vi "Parallel Process Template (JKI-QSM).vi"() -> ()   [LabVIEW 2011, in "Messenging.lvlib" / "Parallel Process Template (JKI-QSM).lvclass"]
uses:
  Parallel Process Template (JKI-QSM).lvclass
  Interprocess Messenger/TextVarientMessage/Write VarMessage.vi
  Interprocess Messenger/VarMessage/VarMessage.lvclass
  Interprocess Messenger/TextVarientMessage/MSG.lvclass
  Parallel Process.lvclass
  Interprocess Messenger/TextVarientMessage/Write (no data).vi
  Interprocess Messenger/EventMessenger/EventMessenger.lvclass
  ObserverRegister/ObserverRegistry.lvclass
  Interprocess Messenger/ErrorMessage/Write ErrorMessage.vi
  Interprocess Messenger/ErrorMessage/ErrorMessage.lvclass
  Interprocess Messenger/TextVarientMessage/Reply (message).vi
panel:
  in  "Startup Message":refnum<class "MSG.lvclass">
  out "current time":timestamp
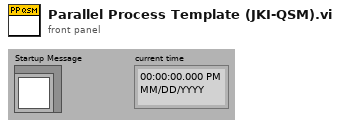
[diagram p1: front panel]
types:
  T1 = enum32{"invalid app kind", "Development System", "Run Time System", "Student Edition", "Embedded LabVIEW", "Evaluation", "Custom"}
  T2 = enum32{"Invalid", "Standard", "Closed", "Hidden", "Minimized", "Maximized"}
  T3 = cluster{"Core":cluster{"Current VI Reference":refnum<vi>, "Close Panel on Exit?":bool}, "Message":refnum<class "MSG.lvclass">, "事件注册引用句柄":refnum<event-registration>}
  T4 = cluster{"Current VI Reference":refnum<vi>, "Close Panel on Exit?":bool}
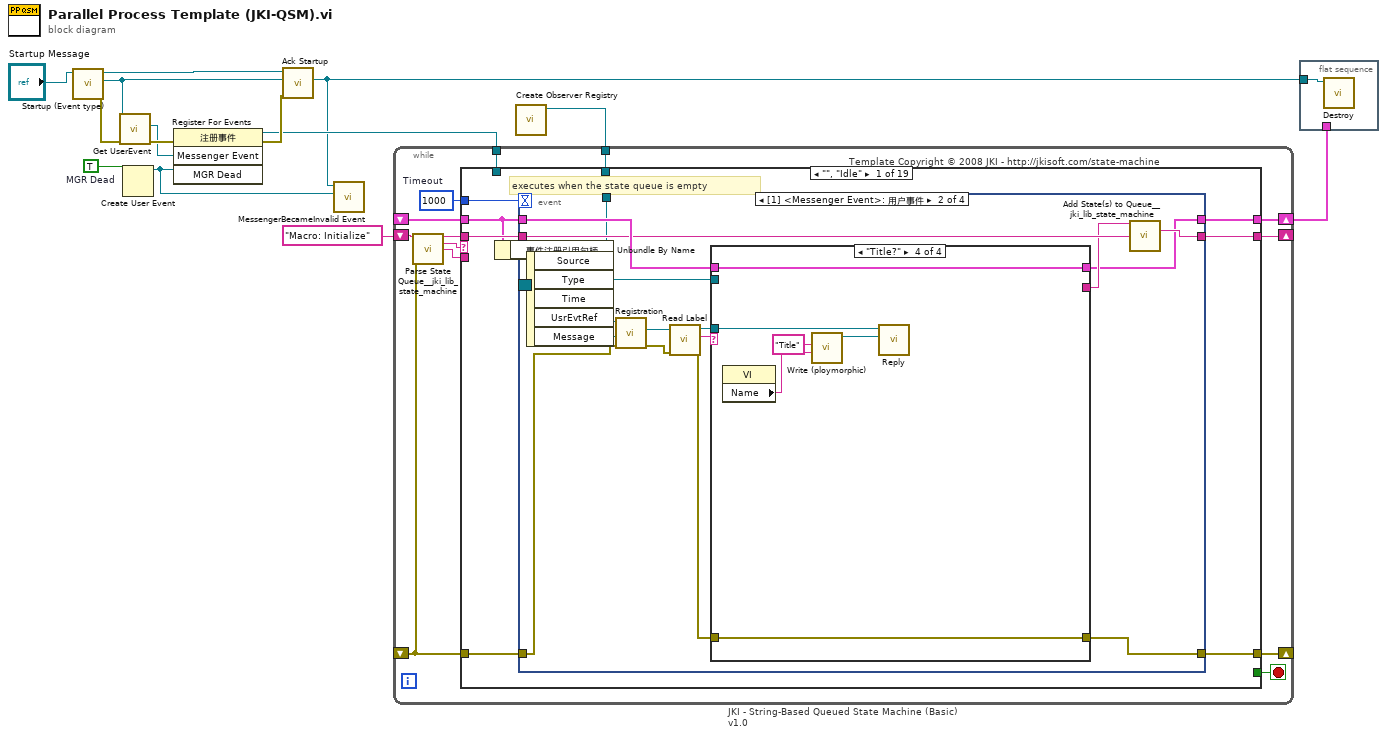
[diagram p0: block diagram]
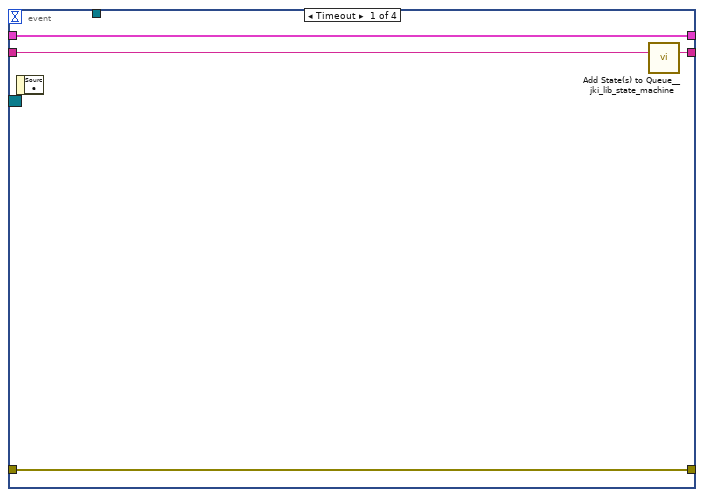
[diagram p2: hidden frame]
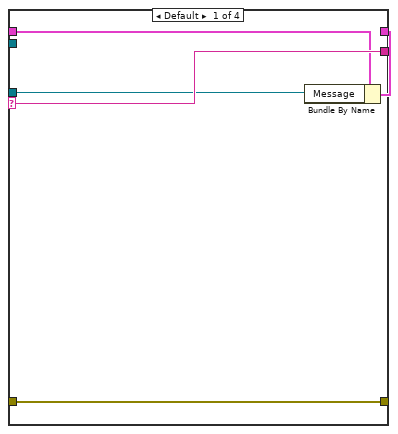
[diagram p3: hidden frame]
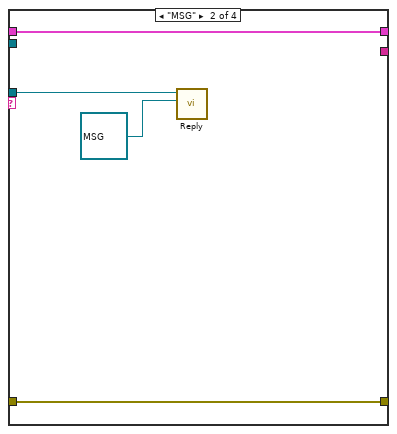
[diagram p4: hidden frame]
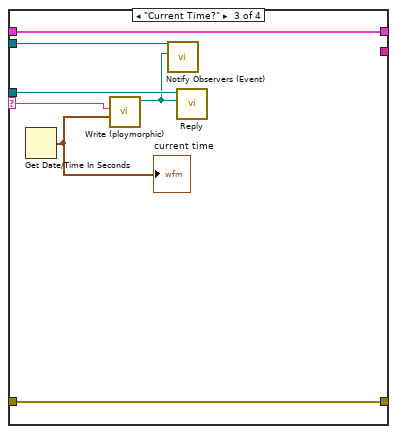
[diagram p5: hidden frame]
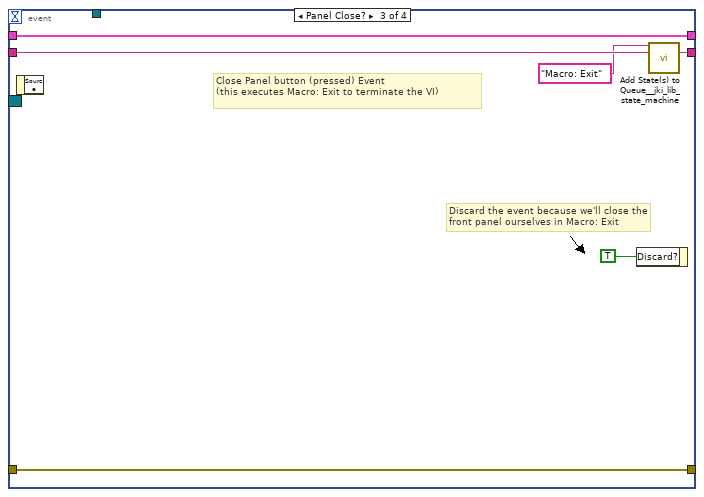
[diagram p6: hidden frame]
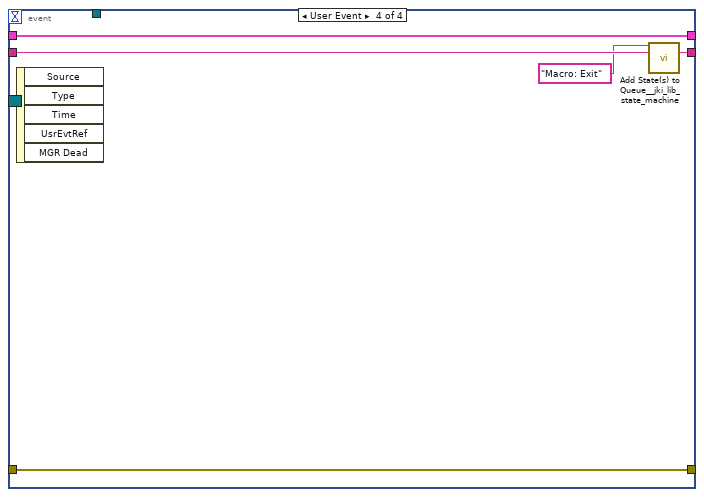
[diagram p7: hidden frame]
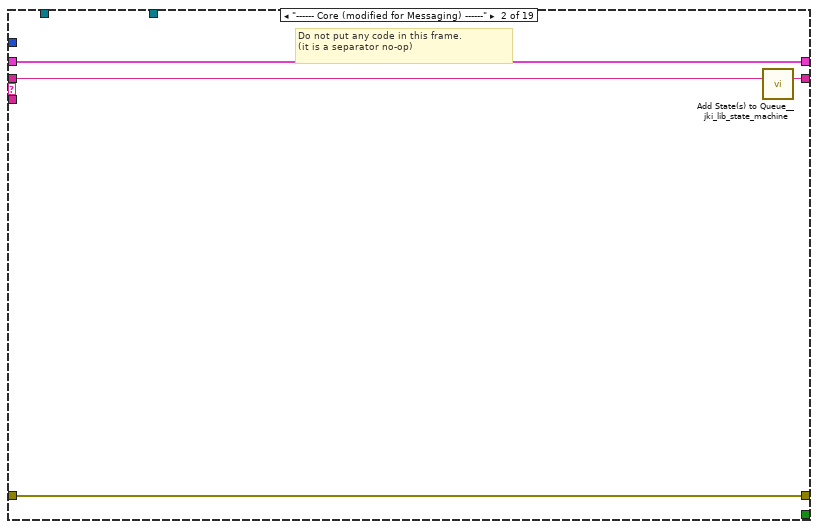
[diagram p8: hidden frame]
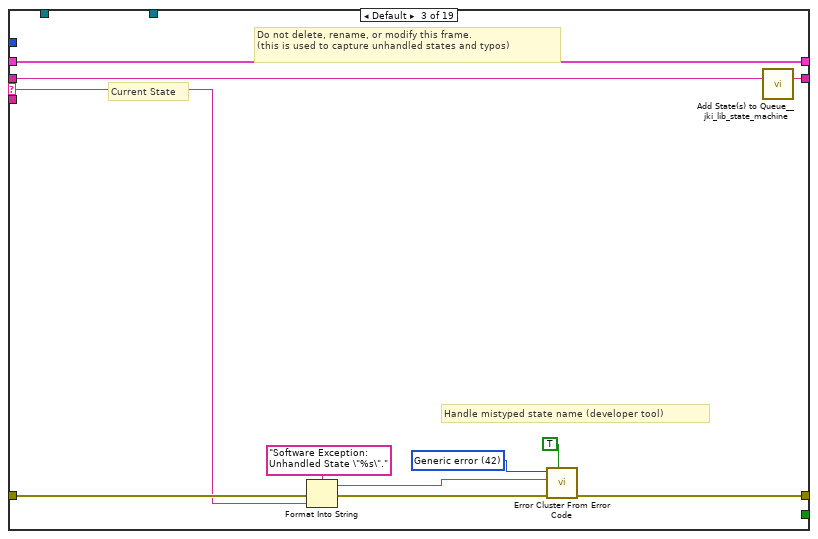
[diagram p9: hidden frame]
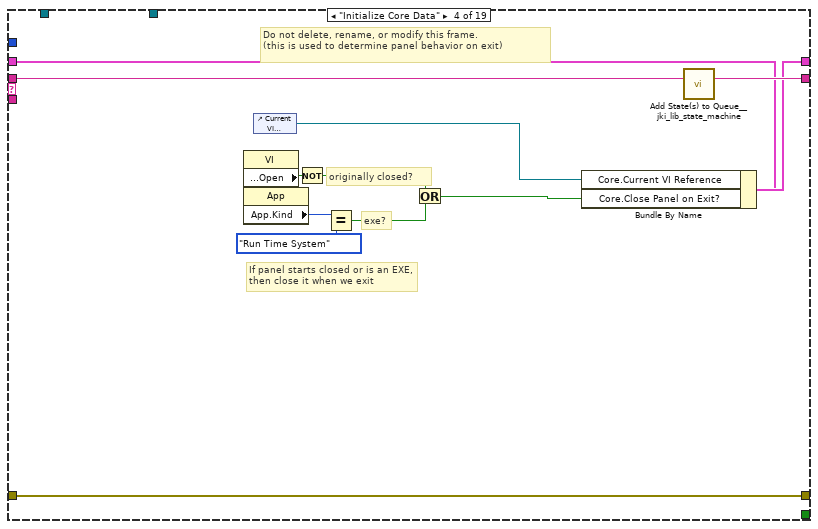
[diagram p10: hidden frame]
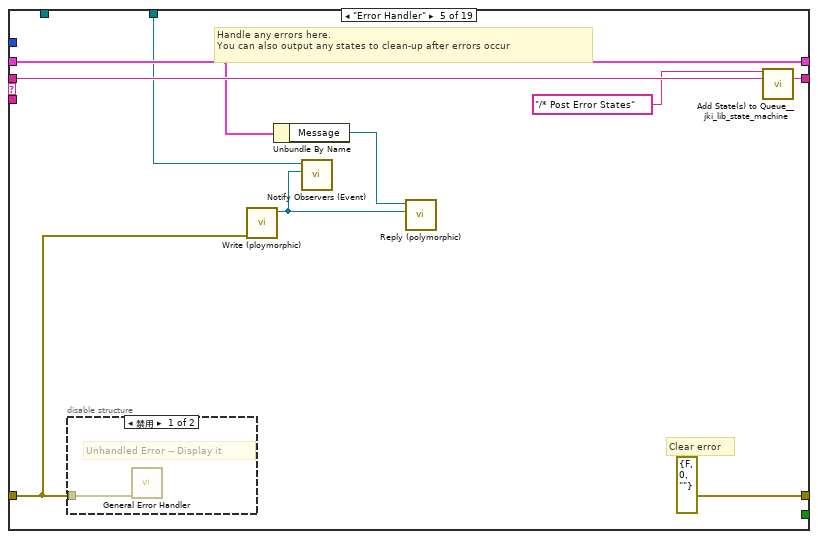
[diagram p11: hidden frame]
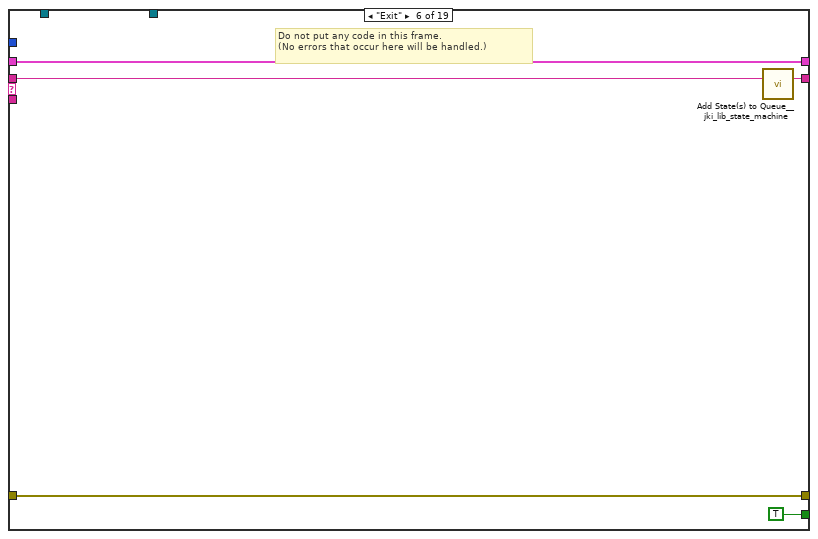
[diagram p13: hidden frame]
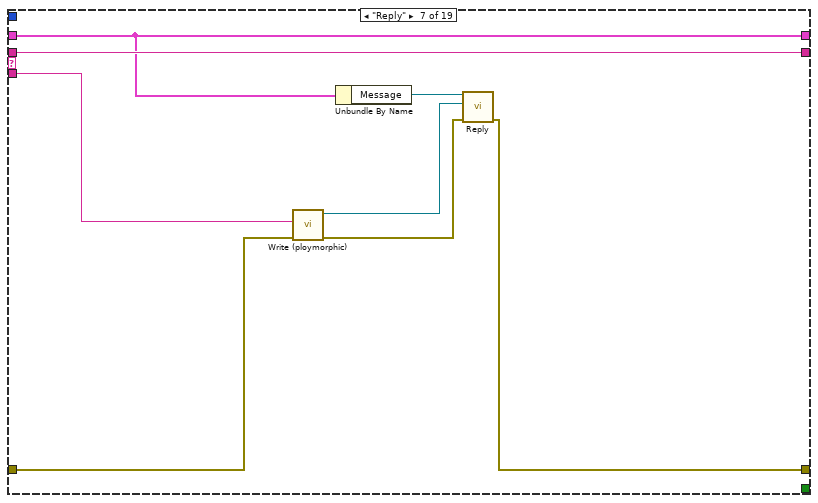
[diagram p14: hidden frame]
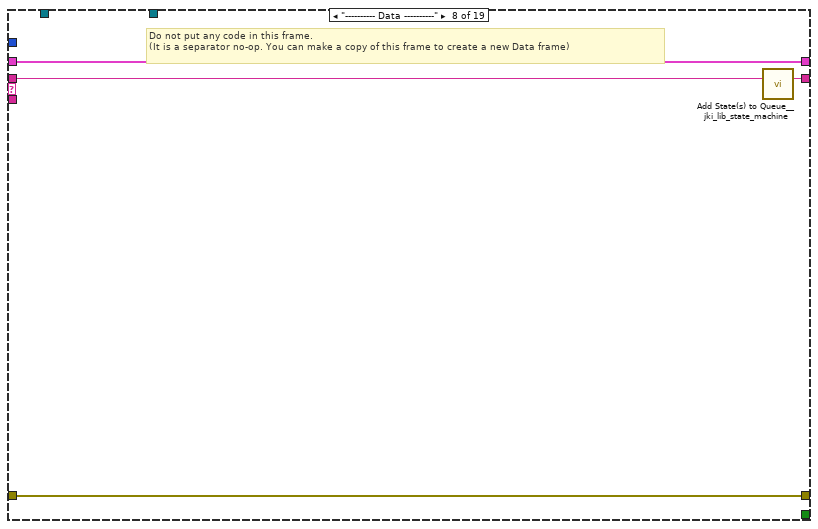
[diagram p15: hidden frame]
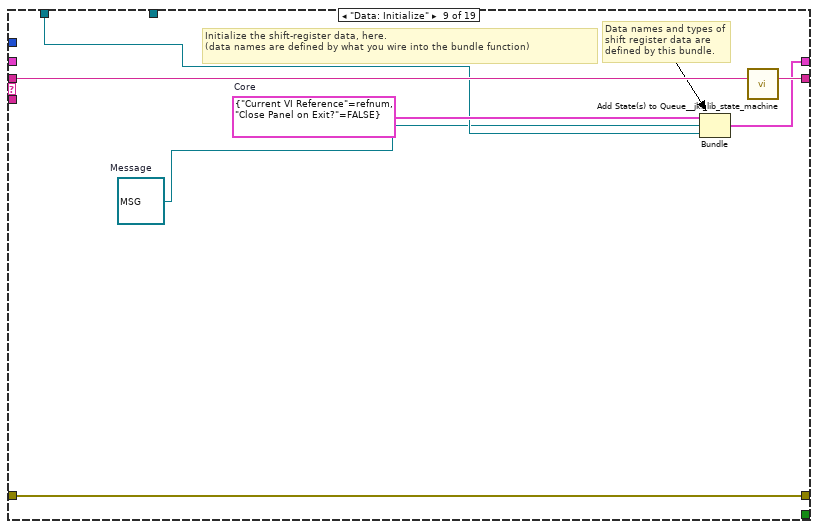
[diagram p16: hidden frame]
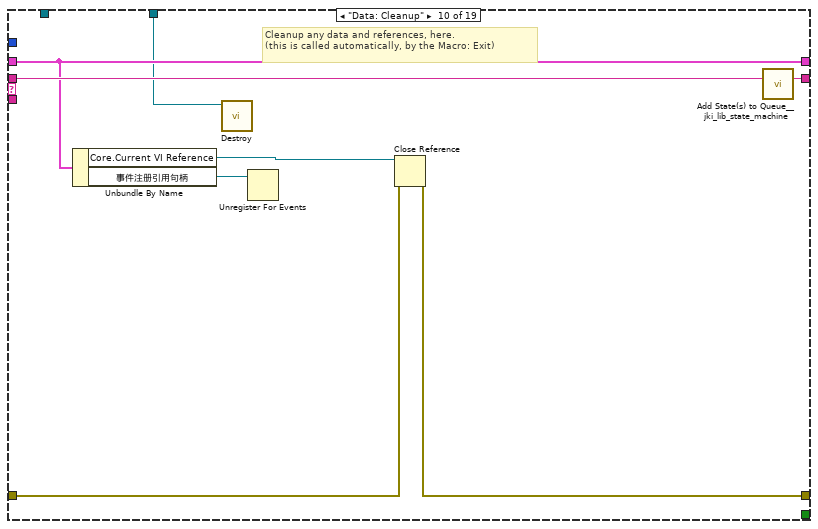
[diagram p17: hidden frame]
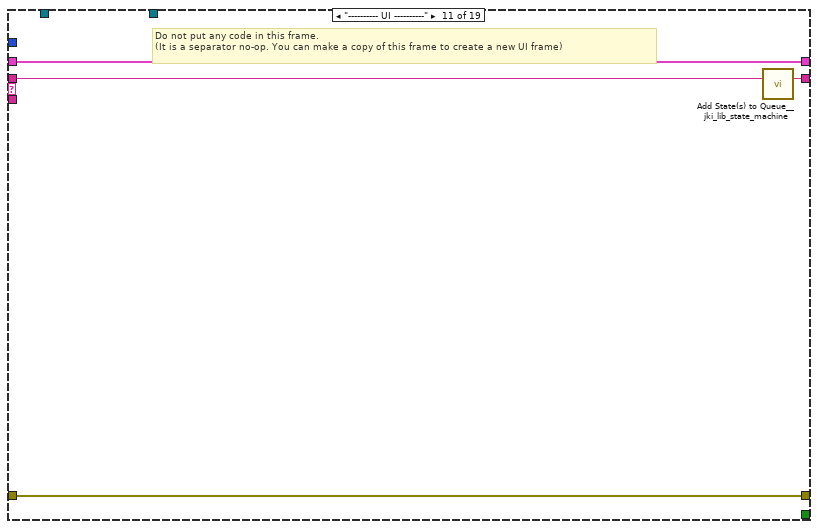
[diagram p18: hidden frame]
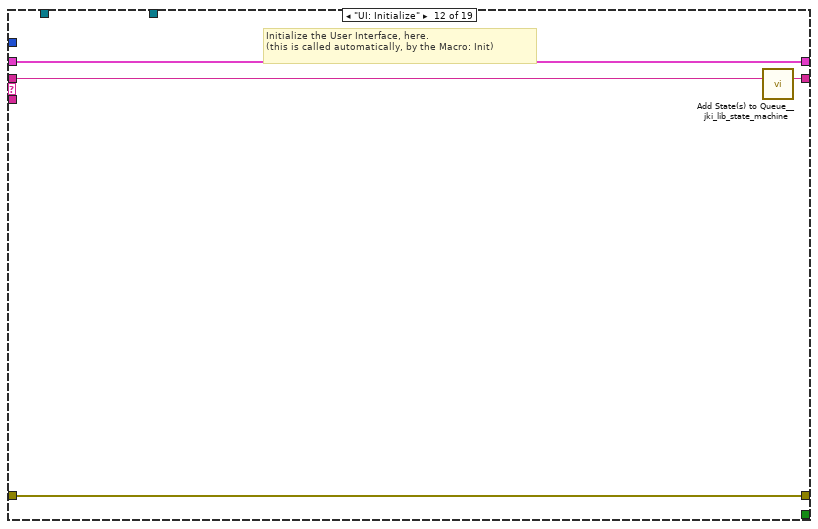
[diagram p19: hidden frame]
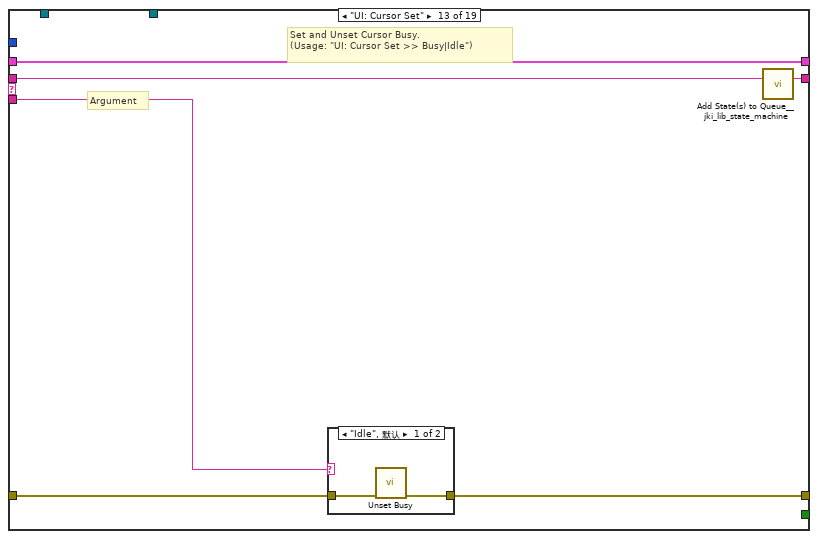
[diagram p20: hidden frame]
diagram:
  w8 = TRUE  # MGR Dead
  n1 = call "Startup (Event type).vi"("Startup Message"="Startup Message") -> ("error out"=w11:errorcluster, "Command Messenger out"=w13:refnum<class "EventMessenger.lvclass">, "Starup Message"=w12:refnum<class "MSG.lvclass">)  [unwired: 2 in, 6 out]
  n2 = call-dynamic "Get UserEvent.vi"("error in"=w11, "EventMessenger"=w13) -> ("error out"=w10:errorcluster, "Messenger Event"=w9:refnum<user-event>)  [unwired: 8 out]
  n3 = Create User Event(user event datatype=w8) -> (user event=w6:refnum<user-event>)  [unwired: 1 in, 1 out]
  n4 = register-events(error in=w10, w9, w6) -> (reference out=w5:refnum<event-registration>, error out=w7:errorcluster)  [unwired: 1 in]
  n5 = call "Ack Startup.vi"("error in"=w7, "Command Messenger"=w13, "Starup Message"=w12) -> ("Command Messenger"=w4:refnum<class "EventMessenger.lvclass">)  [unwired: 3 in, 5 out]
  n6 = call "MessengerBecameInvalid Event.vi"("MGR became Invalid"=w6, "Messenger"=w4) -> ()  [unwired: 1 in, 9 out]
  n7 = call "Create Observer Registry.vi"() -> ("ObsReg"=w1:refnum<class "ObserverRegistry.lvclass">)  [unwired: 1 in, 10 out]
  n8 = while "JKI - String-Based Queued State Machine (Basic) v1.0" {
    shift-right: [w20] -> w3
    shift-left: _ -> [w19]
    shift-right: [w23] -> _
    shift-left: _ -> [w17]
    shift-right: [w22] -> _
    shift-left: "Macro: Initialize" -> [w24]
    tunnel: w5 -> [w16]
    tunnel: w1 -> [w15]
    stop <- w21 stop-if-true
    w18 = 1000  # Timeout
    # "Template Copyright © 2008 JKI - http://jkisoft.com/state-machine"
    n9 = call <vilib>:"Parse State Queue__jki_lib_state_machine.vi"("State Queue"=w24, "Error In (no error)"=w17) -> ("Remaining States"=w26:string, "Current State"=w27:string, "Arguments"=w25:string)  [unwired: 1 in, 10 out]
    n10 = case shown="\"\", \"Idle\"" w27 {
      selector: w27 -> [_ _ w95 _ _ _ _ _ _ _ _ _ _ _ _ _ w215 _ _]
      tunnel: w26 -> [w36 w91 w98 w114 w123 w129 w137 w141 w148 w156 w160 w164 w170 w181 w207 w212 w225 w229 w233]
      tunnel: w25 -> [_ _ _ _ _ _ w130 _ _ _ _ _ w165 w175 _ _ _ _ _]
      tunnel: w19 -> [w30 w88 w94 w105 w119 w127 w133 w138 _ w151 w157 w162 w168 w177 w204 w209 w216 w226 w230]
      tunnel: [w34 w89 w92 w111 errorcluster {"status"=FALSE, "code"=0, "source"=""} ("error out") w126 w131 w139 w145 w152 w158 w161 w166 w178 w205 w210 w223 w227 w231] -> w23
      tunnel: w17 -> [w33 w89 w99 w111 w118 w126 w132 w139 w145 w153 w158 w161 w167 w179 w205 w210 w223 w227 w231]
      tunnel: [w35 w90 w97 w113 w122 w128 w137 w140 w147 w155 w159 w163 w169 w180 w206 w211 w224 w228 w232] -> w22
      tunnel: [_ _ _ _ _ TRUE _ _ _ _ _ _ _ _ _ _ _ _ _] -> w21
      tunnel: [w32 w88 w94 w112 w119 w127 w133 w138 w146 w151 w157 w162 w168 w177 w204 w209 w216 w226 w230] -> w20
      tunnel: w18 -> [w31 _ _ _ _ _ _ _ _ _ _ _ _ _ _ _ _ _ _]
      tunnel: w16 -> [_ _ _ _ _ _ _ _ w143 _ _ _ _ _ _ _ _ _ _]
      tunnel: w15 -> [w28 _ _ _ w116 _ _ _ _ w149 _ _ _ _ _ _ w213 _ _]
      frame "", "Idle" {
        # "executes when the state queue is empty"
        n11 = Unbundle By Name(w30) -> ("事件注册引用句柄"=w29:refnum<event-registration>)
        n12 = event shown="[1] <Messenger Event>: 用户事件" {
          selector: w29 -> [_ _ _ _]
          dyn-events: _ -> [_ _ _ _]
          timeout: w31 -> [_ _ _ _]
          tunnel: w36 -> [w40 w50 w82 w87]
          tunnel: [w39 w54 w81 w86] -> w35
          tunnel: w30 -> [w37 w53 w79 w84]
          tunnel: [w38 w47 w80 w85] -> w34
          tunnel: w33 -> [w38 w43 w80 w85]
          tunnel: [w37 w48 w79 w84] -> w32
          tunnel: w28 -> [_ w41 _ _]
          event Timeout {
            n13 = event-data() -> ()  [unwired: 2 out]
            n14 = call <vilib>:"Add State(s) to Queue__jki_lib_state_machine.vi"("State(s) in (\"\")"=w40) -> ("States Out"=w39:string)  [unwired: 2 in, 12 out]
          }
          event User Event {
            n15 = event-data() -> ("Message"=w45:refnum<class "MSG.lvclass">)  [unwired: 5 out]
            n16 = call "Registration.vi"("error in (no error)"=w43, "Message"=w45, "ObserverRegistry in"=w41) -> ("error out"=w42:errorcluster, "Message (Register Commands filtered out)"=w44:refnum<class "MSG.lvclass">)  [unwired: 7 out]
            n17 = call-dynamic "Read Label.vi"("error in (no error)"=w42, "Message"=w44) -> ("error out"=w46:errorcluster, "Label"=w52:string, "Message"=w51:refnum<class "MSG.lvclass">)  [unwired: 7 out]
            n18 = case shown="\"Title?\"" w52 {
              selector: w52 -> [w59 _ w68 _]
              tunnel: [w59 _ _ _] -> w49
              tunnel: w53 -> [w58 w63 w70 w76]
              tunnel: [w57 w63 w70 w76] -> w48
              tunnel: w51 -> [w56 w62 w69 w75]
              tunnel: w46 -> [w55 w60 w66 w73]
              tunnel: [w55 w60 w66 w73] -> w47
              tunnel: w41 -> [_ _ w65 _]
              frame Default {
                n19 = Bundle By Name(cluster=w58, "Message"=w56) -> (w57:T3)
              }
              frame "MSG" {
                n20 = call-dynamic "Reply.vi"("Reply"=refnum<class "MSG.lvclass"> refnum, "Message to Reply to"=w62) -> ()  [unwired: 1 in, 9 out]
              }
              frame "Current Time?" {
                n21 = Get Date/Time In Seconds() -> (seconds since 1Jan1904=w67:timestamp)
                "current time" <- w67
                n22 = call-poly "Write (ploymorphic).vi"("Varient"=w67, "Label"=w68) -> ("Message"=w64:refnum<class "VarMessage.lvclass">)  [unwired: 1 in, 8 out]
                n23 = call "Notify Observers (Event).vi"("Message"=w64, "ObserverRegistry in"=w65) -> ()  [unwired: 1 in, 9 out]
                n24 = call-dynamic "Reply.vi"("Reply"=w64, "Message to Reply to"=w69) -> ()  [unwired: 1 in, 9 out]
              }
              frame "Title?" {
                n25 = property class="VI"() -> ("Name"=w72:string)  [unwired: 2 in, 2 out]
                n26 = call-poly "Write (ploymorphic).vi"("Varient"=w72, "Label"="Title") -> ("Message"=w74:refnum<class "VarMessage.lvclass">)  [unwired: 1 in, 8 out]
                n27 = call-dynamic "Reply.vi"("Reply"=w74, "Message to Reply to"=w75) -> ()  [unwired: 1 in, 9 out]
              }
            }
            n28 = call <vilib>:"Add State(s) to Queue__jki_lib_state_machine.vi"("State(s) in Front (\"\")"=w49, "State(s) at Back (\"\")"=w50) -> ("States Out"=w54:string)  [unwired: 1 in, 12 out]
          }
          event Panel Close? {
            # "Discard the event because we'll close the front panel ourselves in Macro: Exit"
            # "Close Panel button (pressed) Event\n(this executes Macro: Exit to terminate the VI)"
            n29 = event-data() -> ()  [unwired: 2 out]
            n30 = event-data("Discard?"=TRUE) -> ()  [unwired: 1 in, 1 out]
            n31 = call <vilib>:"Add State(s) to Queue__jki_lib_state_machine.vi"("State(s) in Front (\"\")"="Macro: Exit", "State(s) in (\"\")"=w82) -> ("States Out"=w81:string)  [unwired: 1 in, 12 out]
          }
          event User Event {
            n32 = event-data() -> ()  [unwired: 6 out]
            n33 = call <vilib>:"Add State(s) to Queue__jki_lib_state_machine.vi"("State(s) in Front (\"\")"="Macro: Exit", "State(s) in (\"\")"=w87) -> ("States Out"=w86:string)  [unwired: 1 in, 12 out]
          }
        }
      }
      frame "------ Core (modified for Messaging) ------" {
        # "Do not put any code in this frame.\n(it is a separator no-op)"
        n34 = call <vilib>:"Add State(s) to Queue__jki_lib_state_machine.vi"("State(s) in (\"\")"=w91) -> ("States Out"=w90:string)  [unwired: 2 in, 12 out]
      }
      frame Default {
        w101 = 42 items=["No error", "Argument error", "Memory is full", "Out of zone", "End of file", "File already open", "Generic file I/O error", "File not found", "File permission error", "Disk is full", "Duplicate path", "Too many files open", "System feature not enabled", "Resource file not found", "Cannot add resource", "Resource not found", "Image not found", "Image memory error", "Pen does not exist", "Config type invalid", "Config token not found", "Config parse error", "Config memory error", "Bad external code format", "Bad external code offset", "External code not present", "Null window", "Destroy window error", "Null menu", "Print aborted", "Bad print record", "Print driver error", "Windows error during printing", "Memory error during printing", "Print dialog error", "Generic print error", "Invalid device refnum", "Device not found", "Device parameter error", "Device unit error", "Cannot open device", "Device call aborted", "Generic error", "Cancelled by user", "Object ID too low", "Object ID too high", "Object not in heap", "Unknown heap", "Unknown object (invalid DefProc)", "Unknown object (DefProc not in table)", "Message out of range", "Invalid (null) method", "Unknown message", "Manager call not supported", "Bad address", "Network operation in progress", "Network operation timed out", "Connection is busy", "Network attribute not supported", "Network error", "Address in use", "System out of memory", "Connection aborted", "Connection refused", "Not connected", "Already connected", "Connection closed", "Initialization error (interapplication manager)", "Bad occurrence", "Wait on unbound occurrence handler", "Occurrence queue overflow", "Datalog type conflict", "Unused", "Unrecognized type (interapplication manager)", "Memory corrupt", "Failed to make temporary DLL", "Old CIN version", "Drag socket not found", "Failed to load drop-object", "Failed to register OLE object", "Failed to release OLE object", "Format specifier type mismatch", "Unknown format specifier", "Too few format specifiers", "Too many format specifiers", "Scan failed", "Newer CIN version", "Error converting to variant", "Runtime menu error", "Password tampered", "Variant attribute not found", "Incompatible variant data type", "Event data is not available", "Event Store is not present", "Occurrence is not found", "Event Queue is not created", "Event info is not available", "Refnum passed is NULL", "Error retrieving Class GUID", "Error retrieving CoClass GUID", "Error retrieving TypeLib GUID.", "Bad built application magic bytes.", "Specific driver is different from the specific driver associated with the Logical Name.", "There is no session opened to the class driver.", "Max Error", "MAX - Error with config objects", "MAX - Error loading configuration", "MAX - Group not supported"]
        # "Current State"
        # "Do not delete, rename, or modify this frame.\n(this is used to capture unhandled states and typos)"
        # "Handle mistyped state name (developer tool)"
        n35 = Format Into String(format string="Software Exception: Unhandled State \"%s\"." ("message"), error in=w99, w95) -> (resulting string=w93:string, error out=w100:errorcluster)  [unwired: 1 in]
        n36 = call <vilib>:"Error Cluster From Error Code.vi"("show call chain? (False)"=TRUE, "error in (no error)"=w100, "error message (\"\")"=w93, "error code (0)"=w101) -> ("error out"=w92:errorcluster)  [unwired: 5 out]
        n37 = call <vilib>:"Add State(s) to Queue__jki_lib_state_machine.vi"("State(s) in (\"\")"=w98) -> ("States Out"=w97:string)  [unwired: 2 in, 12 out]
      }
      frame "Initialize Core Data" {
        # "Do not delete, rename, or modify this frame.\n(this is used to determine panel behavior on exit)"
        # "originally closed?"
        # "exe?"
        # "If panel starts closed or is an EXE, then close it when we exit"
        n38 = property class="VI"() -> ("Front Panel.Open"=w110:bool)  [unwired: 2 in, 2 out]
        n39 = property class="App"() -> ("App.Kind"=w109:T1)  [unwired: 2 in, 2 out]
        n40 = control-ref of="Current VI Reference"() -> (w103:refnum<vi>)
        n41 = Not(x=w110) -> (.not. x?=w107:bool)
        n42 = Equal?(x=w109, y=T1."Run Time System" ("Application:Kind")) -> (x = y?=w106:bool)
        n43 = Or(x=w107, y=w106) -> (x .or. y?=w104:bool)
        n44 = Bundle By Name(cluster=w105, "Core.Current VI Reference"=w103, "Core.Close Panel on Exit?"=w104) -> (w112:T3)
        n45 = call <vilib>:"Add State(s) to Queue__jki_lib_state_machine.vi"("State(s) in (\"\")"=w114) -> ("States Out"=w113:string)  [unwired: 2 in, 12 out]
      }
      frame "Error Handler" {
        # "Handle any errors here.\nYou can also output any states to clean-up after errors occur"
        # "Clear error"
        n46 = disable-structure shown="禁用" {
          disable-tunnel: w118 -> [w124 _]
          frame Disabled {
            # "Unhandled Error -- Display it"
            n47 = call <vilib>:"General Error Handler.vi"("error in (no error)"=w124) -> ()  [unwired: 1 in, 14 out]
          }
          frame Enabled {
          }
        }
        n48 = call-poly "Write (ploymorphic).vi"("error (to be sent)"=w118) -> ("Message"=w115:refnum<class "ErrorMessage.lvclass">)  [unwired: 1 in, 9 out]
        n49 = Unbundle By Name(w119) -> ("Message"=w117:refnum<class "MSG.lvclass">)
        n50 = call "Notify Observers (Event).vi"("Message"=w115, "ObserverRegistry in"=w116) -> ()  [unwired: 1 in, 9 out]
        n51 = call-poly "Reply (polymorphic).vi"("Reply"=w115, "Message to Reply to"=w117) -> ()  [unwired: 1 in, 9 out]
        n52 = call <vilib>:"Add State(s) to Queue__jki_lib_state_machine.vi"("State(s) in Front (\"\")"="/* Post Error States", "State(s) in (\"\")"=w123) -> ("States Out"=w122:string)  [unwired: 1 in, 12 out]
      }
      frame "Exit" {
        # "Do not put any code in this frame.\n(No errors that occur here will be handled.)"
        n53 = call <vilib>:"Add State(s) to Queue__jki_lib_state_machine.vi"("State(s) in (\"\")"=w129) -> ("States Out"=w128:string)  [unwired: 2 in, 12 out]
      }
      frame "Reply" {
        n54 = call-poly "Write (ploymorphic).vi"("error in (no error)"=w132, "Label"=w130) -> ("error out"=w134:errorcluster, "Message"=w135:refnum<class "MSG.lvclass">)  [unwired: 8 out]
        n55 = Unbundle By Name(w133) -> ("Message"=w136:refnum<class "MSG.lvclass">)
        n56 = call-dynamic "Reply.vi"("error in (no error)"=w134, "Reply"=w135, "Message to Reply to"=w136) -> ("error out"=w131:errorcluster)  [unwired: 8 out]
      }
      frame "---------- Data ----------" {
        # "Do not put any code in this frame.\n(It is a separator no-op. You can make a copy of this frame to create a new Data frame)"
        n57 = call <vilib>:"Add State(s) to Queue__jki_lib_state_machine.vi"("State(s) in (\"\")"=w141) -> ("States Out"=w140:string)  [unwired: 2 in, 12 out]
      }
      frame "Data: Initialize" {
        w142 = refnum<class "MSG.lvclass"> refnum  # Message
        w144 = T4 {"Current VI Reference"=refnum, "Close Panel on Exit?"=FALSE}  # Core
        # "Data names and types of shift register data are defined by this bundle."
        # "Initialize the shift-register data, here.\n(data names are defined by what you wire into the bundle function)"
        n58 = Bundle("Core"=w144, "Message"=w142, "事件注册引用句柄"=w143) -> (w146:T3)  [unwired: 1 out]
        n59 = call <vilib>:"Add State(s) to Queue__jki_lib_state_machine.vi"("State(s) in (\"\")"=w148) -> ("States Out"=w147:string)  [unwired: 2 in, 12 out]
      }
      frame "Data: Cleanup" {
        # "Cleanup any data and references, here.\n(this is called automatically, by the Macro: Exit)"
        n60 = Unbundle By Name(w151) -> ("Core.Current VI Reference"=w154:refnum<vi>, "事件注册引用句柄"=w150:refnum<event-registration>)
        n61 = call "Destroy.vi"("ObserverRegistry.lvclass in"=w149) -> ()  [unwired: 1 in, 10 out]
        n62 = Unregister For Events(event registration refnum=w150) -> ()  [unwired: 1 in, 1 out]
        n63 = Close Reference(reference=w154, error in (no error)=w153) -> (error out=w152:errorcluster)
        n64 = call <vilib>:"Add State(s) to Queue__jki_lib_state_machine.vi"("State(s) in (\"\")"=w156) -> ("States Out"=w155:string)  [unwired: 2 in, 12 out]
      }
      frame "---------- UI ----------" {
        # "Do not put any code in this frame.\n(It is a separator no-op. You can make a copy of this frame to create a new UI frame)"
        n65 = call <vilib>:"Add State(s) to Queue__jki_lib_state_machine.vi"("State(s) in (\"\")"=w160) -> ("States Out"=w159:string)  [unwired: 2 in, 12 out]
      }
      frame "UI: Initialize" {
        # "Initialize the User Interface, here.\n(this is called automatically, by the Macro: Init)"
        n66 = call <vilib>:"Add State(s) to Queue__jki_lib_state_machine.vi"("State(s) in (\"\")"=w164) -> ("States Out"=w163:string)  [unwired: 2 in, 12 out]
      }
      frame "UI: Cursor Set" {
        # "Argument"
        # "Set and Unset Cursor Busy.\n(Usage: \"UI: Cursor Set >> Busy|Idle\")"
        n67 = case shown="\"Idle\", 默认" w165 {
          tunnel: w167 -> [w172 w174]
          tunnel: [w171 w173] -> w166
          frame "Idle", Default {
            n68 = call <vilib>:"Unset Busy.vi"("error in (no error)"=w172) -> ("error out"=w171:errorcluster)  [unwired: 1 in, 9 out]
          }
          frame "Busy" {
            n69 = call <vilib>:"Set Busy.vi"("error in (no error)"=w174) -> ("error out"=w173:errorcluster)  [unwired: 3 in, 7 out]
          }
        }
        n70 = call <vilib>:"Add State(s) to Queue__jki_lib_state_machine.vi"("State(s) in (\"\")"=w170) -> ("States Out"=w169:string)  [unwired: 2 in, 12 out]
      }
      frame "UI: Front Panel State" {
        # "Argument"
        # "Set Front Panel Open or Closed\n(Usage: \"UI: Front Panel State >> Open|Close\")"
        n71 = Unbundle By Name(w177) -> ("Core.Current VI Reference"=w176:refnum<vi>)
        n72 = case shown="\"Open\", 默认" w175 {
          tunnel: w179 -> [w185 w198]
          tunnel: [w187 w199] -> w178
          tunnel: w176 -> [w186 w196]
          frame "Open", Default {
            n73 = property class="VI"(reference=w186, error in=w185) -> (reference out=w183:refnum<vi>, error out=w184:errorcluster, "Front Panel.Open"=w182:bool)
            n74 = case shown="假" w182 {
              tunnel: [w190 w193] -> w187
              tunnel: w184 -> [w189 w193]
              tunnel: w183 -> [w188 _]
              frame False {
                n75 = invoke class="VI" method="FP.Open"(reference=w188, error in=w189, "Activate"=TRUE, "State"=T2."Standard") -> (error out=w190:errorcluster)  [unwired: 1 in, 4 out]
              }
              frame True {
              }
            }
          }
          frame "Close" {
            n76 = property class="VI"(reference=w196, error in=w198) -> (reference out=w195:refnum<vi>, error out=w197:errorcluster, "Front Panel.Open"=w194:bool)
            n77 = case shown="真" w194 {
              tunnel: [w200 w203] -> w199
              tunnel: w197 -> [w200 w202]
              tunnel: w195 -> [_ w201]
              frame False {
              }
              frame True {
                n78 = invoke class="VI" method="FP.Close"(reference=w201, error in=w202) -> (error out=w203:errorcluster)  [unwired: 1 in, 2 out]
              }
            }
          }
        }
        n79 = call <vilib>:"Add State(s) to Queue__jki_lib_state_machine.vi"("State(s) in (\"\")"=w181) -> ("States Out"=w180:string)  [unwired: 2 in, 12 out]
      }
      frame "---------- Macro ----------" {
        # "Do not put any code in this frame.\n(It is a separator no-op. You can make a copy of this frame to create a new Macro frame)"
        n80 = call <vilib>:"Add State(s) to Queue__jki_lib_state_machine.vi"("State(s) in (\"\")"=w207) -> ("States Out"=w206:string)  [unwired: 2 in, 12 out]
      }
      frame "Macro: Initialize" {
        w208 = "Data: Initialize\nInitialize Core Data\nUI: Initialize\n// UI: Front Panel State >> Open"  # Data: Initialize Initialize Core Data UI: Initialize // UI: Front Panel State >> Open
        # "Initialization Macro\n(This is called once, when the VI starts)"
        n81 = call <vilib>:"Add State(s) to Queue__jki_lib_state_machine.vi"("State(s) in Front (\"\")"=w208, "State(s) in (\"\")"=w212) -> ("States Out"=w211:string)  [unwired: 1 in, 12 out]
      }
      frame "Macro: Exit" {
        # "Exit Macro\n(This is called once, when the VI exits)"
        n82 = Unbundle By Name(w216) -> ("Core.Close Panel on Exit?"=w222:bool)
        n83 = call-poly "Write (ploymorphic).vi"("Label"=w215) -> ("Message"=w214:refnum<class "MSG.lvclass">)  [unwired: 1 in, 9 out]
        n84 = call "Notify Observers (Event).vi"("Message"=w214, "ObserverRegistry in"=w213) -> ()  [unwired: 1 in, 9 out]
        n85 = Select(t="UI: Front Panel State >> Close", s=w222, f="") -> (s? t:f=w219:string)
        n86 = call <vilib>:"Add State(s) to Queue__jki_lib_state_machine.vi"("State(s) in (\"\")"=w219, "State(s) at Back (\"\")"="PP: Reply >> Shutdown\nData: Cleanup\nExit") -> ("States Out"=w217:string)  [unwired: 1 in, 12 out]
        n87 = call <vilib>:"Add State(s) to Queue__jki_lib_state_machine.vi"("State(s) in Front (\"\")"=w217, "State(s) in (\"\")"=w225) -> ("States Out"=w224:string)  [unwired: 1 in, 12 out]
      }
      frame "---------- New Category ----------" {
        # "Template Separator\n(You can make a copy of, or modify, this frame)"
        n88 = call <vilib>:"Add State(s) to Queue__jki_lib_state_machine.vi"("State(s) in (\"\")"=w229) -> ("States Out"=w228:string)  [unwired: 2 in, 12 out]
      }
      frame "New Category: 1" {
        # "Your code here.\n(You can make a copy of, or modify, this frame)"
        n89 = call <vilib>:"Add State(s) to Queue__jki_lib_state_machine.vi"("State(s) in (\"\")"=w233) -> ("States Out"=w232:string)  [unwired: 2 in, 12 out]
      }
    }
  }
  n90 = flat-sequence {
    tunnel: w4 -> [w234]
    tunnel: w3 -> [_]
    frame #0 {
      n91 = call-dynamic "Destroy.vi"("EventMessenger in"=w234) -> ()  [unwired: 1 in, 10 out]
    }
  }
